vi "CamMom.vi"() -> ()   [LabVIEW 2011]
panel:
  out "CameraMom":i32[][](array[numeric])
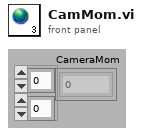
[diagram p1: front panel]
diagram:
